vi "Initialize ActiveX.vi"(6 "Force Init (F)":bool, 7 "FW Unique ID":string="FW1", 8 "error in (no error)":errorcluster, 9 "Mono ID":string, 10 "Unique ID":string="Mono1", 11 "Spectrometer iHR320 In":refnum<class "Spectrometer ActiveX.lvclass">) -> (0 "error out":errorcluster, 1 "FW RefNum Out":refnum<k7>, 2 "Refnum out":refnum<k7> caption="Mono RefNum out", 3 "Spectrometer iHR320 Out":refnum<class "Spectrometer ActiveX.lvclass">)   [LabVIEW 2015, in "Spectrometer ActiveX.lvclass"]
doc: "Initializes a JY Monochromator/Spectrometer based off of its Unique ID (Mono1,Mono2,...) and returns the Reference Number to the associated ActiveX object.\n\nMono ID is an arbitrary name for the spectrometer."
uses:
  Spectrometer ActiveX.lvclass
  Spectrometer ActiveX.lvclass/Spectrometer ActiveX.ctl
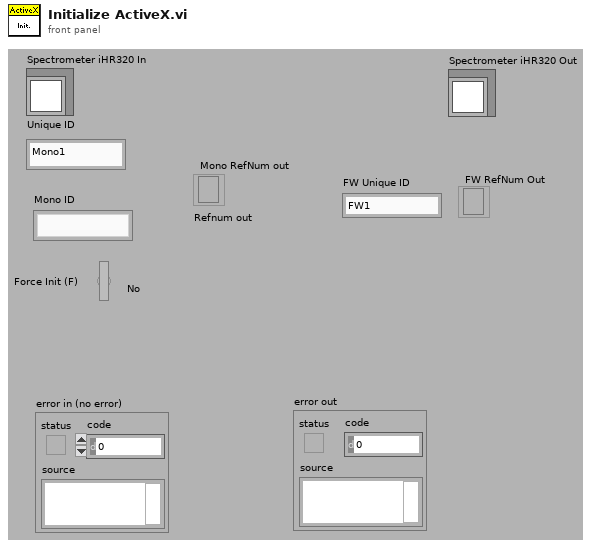
[diagram p1: front panel]
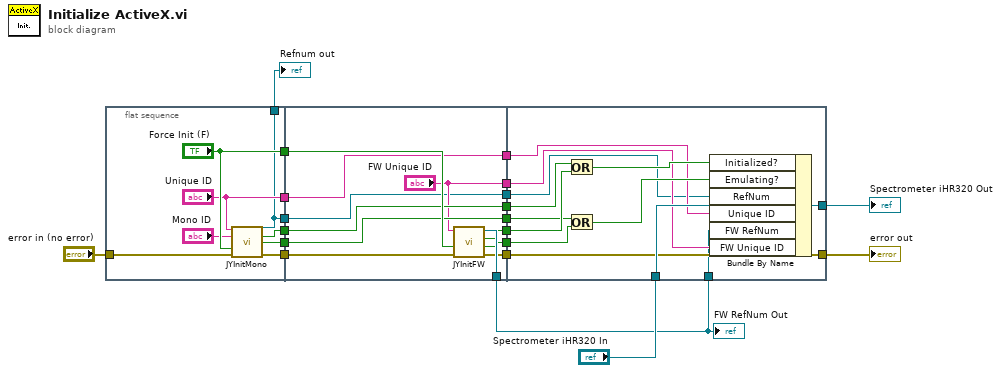
[diagram p0: block diagram]
diagram:
  n1 = flat-sequence {
    tunnel: [w28] -> w18
    tunnel: "error in (no error)" -> [w27]
    tunnel: ["Force Init (F)"] -> w16
    tunnel: [w21] -> w15
    tunnel: [w24] -> w12
    tunnel: [w23] -> w10
    tunnel: ["Unique ID"] -> w4
    tunnel: [w21] -> w2
    tunnel: w18 -> [w39]
    tunnel: w16 -> [w38]
    tunnel: [w37] -> w1
    tunnel: [w36] -> w14
    tunnel: [w35] -> w13
    tunnel: w12 -> [w35]
    tunnel: [w34] -> w11
    tunnel: w10 -> [w34]
    tunnel: [w33] -> w9
    tunnel: [w32] -> w8
    tunnel: ["FW Unique ID"] -> w6
    tunnel: [w30] -> w5
    tunnel: w4 -> [w30]
    tunnel: [w29] -> w3
    tunnel: w2 -> [w29]
    tunnel: "Spectrometer iHR320 In" -> [w52]
    tunnel: [w51] -> w19
    tunnel: w14 -> [w48]
    tunnel: w13 -> [w47]
    tunnel: w11 -> [w46]
    tunnel: w9 -> [w45]
    tunnel: w8 -> [w44]
    tunnel: [w44] -> w7
    tunnel: w6 -> [w43]
    tunnel: w5 -> [w42]
    tunnel: w3 -> [w41]
    tunnel: w1 -> [w40]
    frame #0 {
      n2 = call "JYInitMono.vi"("Unique ID"="Unique ID", "Mono ID"="Mono ID", "Force Init"="Force Init (F)", "error in (no error)"=w27) -> ("Mono RefNum out"=w21:refnum<k7>, "Initialized"=w24:bool, "Emulating"=w23:bool, "error out"=w28:errorcluster)  [unwired: 7 in, 1 out]
    }
    frame #1 {
      n3 = call "JYInitFW.vi"("error in (no error)"=w39, "Force?"=w38, "FW Unique ID"="FW Unique ID") -> ("error out"=w32:errorcluster, "Emulating"=w33:bool, "Initialized"=w36:bool, "FW RefNum Out"=w37:refnum<k7>)  [unwired: 5 in]
    }
    frame #2 {
      n4 = Or(x=w47, y=w48) -> (x .or. y?=w50:bool)
      n5 = Or(x=w46, y=w45) -> (x .or. y?=w49:bool)
      n6 = Bundle By Name(cluster=w52, "Initialized?"=w50, "Emulating?"=w49, "RefNum"=w41, "Unique ID"=w42, "FW RefNum"=w40, "FW Unique ID"=w43) -> (w51:refnum<class "Spectrometer ActiveX.lvclass">)
    }
  }
  "Spectrometer iHR320 Out" <- w19
  "error out" <- w7
  "FW RefNum Out" <- w1
  "Refnum out" <- w15
